vi "Run Bfr Rx - PingPongSized - Check Active.vi"(8 "error in (no error)":errorcluster, 10 "Data in":u8[](array[numeric]), 11 "Ping Pong Buffer in":T1 {"Active Buffer Ref" format="%016x"}) -> (0 "error out":errorcluster, 2 "Data out":u8[](array[numeric]), 3 "Ping Pong Buffer out":T1 {"Active Buffer Ref" format="%016x"}, 4 "Change Active":bool, 6 "Data Size out":u64)   [LabVIEW 2021, in "UDP-Custom-Device Engine.lvlib"]
uses:
  UDP-Custom-Device Engine.lvlib
  Types/Engine - Buffered Rx Ping Pong Buffer.ctl
  Types/Engine - Buffered Rx Active Buffer.ctl
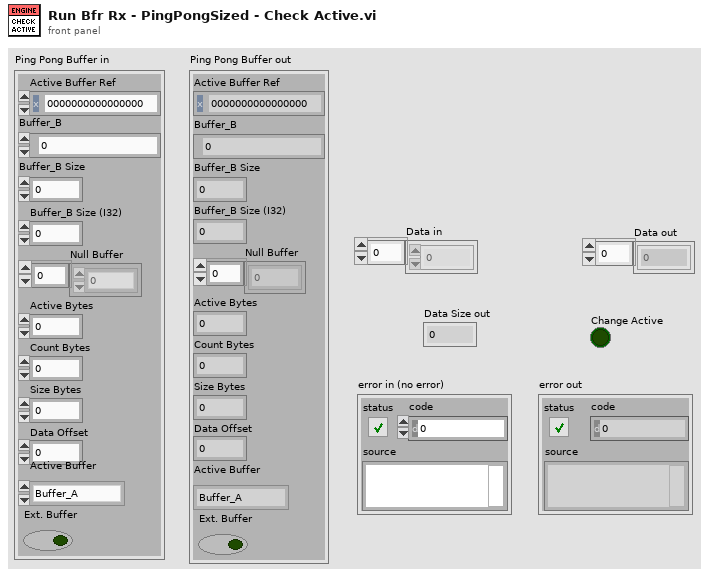
[diagram p1: front panel]
types:
  T1 = typedef "UDP-Custom-Device Engine.lvlib/Engine - Buffered Rx Ping Pong Buffer.ctl" = cluster{"Active Buffer Ref":u64, "Buffer_B":u64, "Buffer_B Size":u64, "Buffer_B Size (I32)":i32, "Null Buffer":u8[], "Active Bytes":u64, "Count Bytes":u64, "Size Bytes":u64, "Data Offset":u64, "Active Buffer":T2, "Ext. Buffer":bool}
  T2 = typedef "UDP-Custom-Device Engine.lvlib/Engine - Buffered Rx Active Buffer.ctl" = enum16{"Buffer_A", "Buffer_B"}
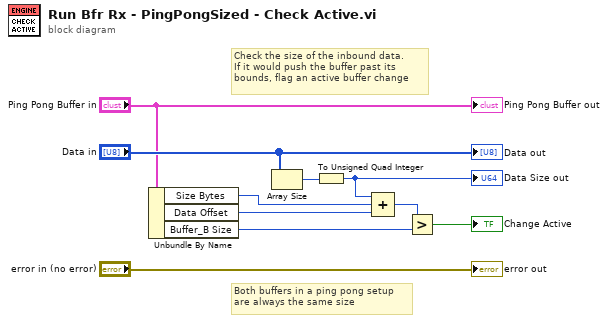
[diagram p0: block diagram]
diagram:
  # "Both buffers in a ping pong setup\nare always the same size"
  # "Check the size of the inbound data.\nIf it would push the buffer past its\nbounds, flag an active buffer change"
  n1 = Unbundle By Name("Ping Pong Buffer in") -> ("Size Bytes"=w1:u64, "Data Offset"=w2:u64, "Buffer_B Size"=w3:u64)
  n2 = Array Size(array="Data in") -> (size(s)=w6:i32)
  n3 = To Unsigned Quad Integer(1:w6) -> (0:w5:u64)
  "Data Size out" <- w5
  n4 = Compound Arithmetic op=ADD(w5, w1, w2) -> (w8:u64)
  n5 = Greater?(x=w8, y=w3) -> (0:→"Change Active":bool)
  "error out" <- "error in (no error)"
  "Data out" <- "Data in"
  "Ping Pong Buffer out" <- "Ping Pong Buffer in"
